vi "Picture_Square_Pixel.vi"(8 "input cluster":T1, 11 "Square":bool) -> (0 "Output Cluster":T1)   [LabVIEW 2009]
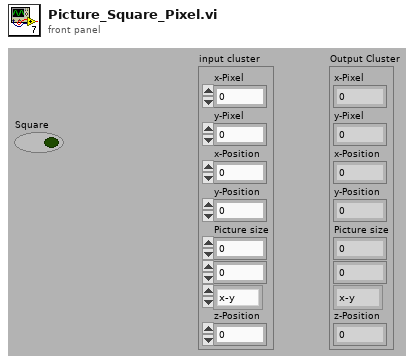
[diagram p1: front panel]
types:
  T1 = cluster{"x-Pixel":u16, "y-Pixel":u16, "x-Position":dbl, "y-Position":dbl, "Picture size":dbl, dbl, enum32{"x-y", "x-z", "y-z"}, "z-Position":dbl}
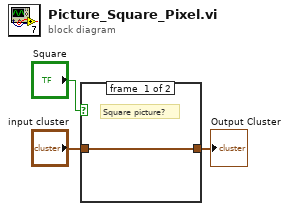
[diagram p0: block diagram]
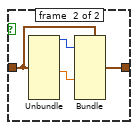
[diagram p2: hidden frame]
diagram:
  n1 = case shown="True" "Square" {
    tunnel: "input cluster" -> [w4 w8]
    tunnel: [w4 w5] -> w1
    frame #0 {
      # "Square picture?"
    }
    frame #1 {
      n2 = Unbundle(w8) -> ("x-Pixel"=w7:u16, "Picture size"=w6:dbl)  [unwired: 6 out]
      n3 = Bundle(cluster=w8, "y-Pixel"=w7, w6) -> (w5:T1)  [unwired: 6 out]
    }
  }
  "Output Cluster" <- w1
